vi "write to build log.vi"(10 "text":string, 11 "log":path) -> ()   [LabVIEW 2013]
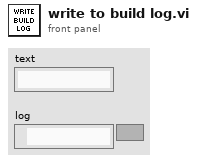
[diagram p1: front panel]
types:
  T1 = enum16{"open", "replace", "create", "open or create", "replace or create", "replace or create with confirmation"}
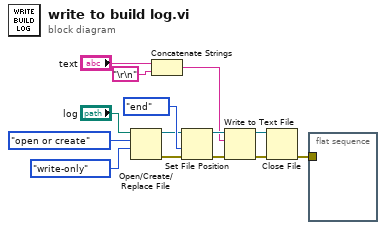
[diagram p0: block diagram]
diagram:
  n1 = Open/Create/Replace File(file path (use dialog)="log", operation (0:open)=T1."open or create", access (0:read/write)=enum16{"read/write", "read-only", "write-only"}."write-only") -> (refnum out=w10:refnum<file>, error out=w3:errorcluster)  [unwired: 3 in, 1 out]
  n2 = Concatenate Strings("text", "\r\n") -> (w2:string)
  n3 = Set File Position(refnum=w10, from (0:start)=enum16{"start", "end", "current"}."end", error in=w3) -> (refnum out=w11:refnum<file>, error out=w9:errorcluster)  [unwired: 1 in]
  n4 = Write to Text File(file (use dialog)=w11, text=w2, error in=w9) -> (refnum out=w4:refnum<file>, error out=w5:errorcluster)  [unwired: 1 in, 1 out]
  n5 = Close File(refnum=w4, error in=w5) -> (error out=w6:errorcluster)  [unwired: 1 out]
  n6 = flat-sequence {
    tunnel: w6 -> [_]
    frame #0 {
    }
  }
